vi "_word.table.Size.vi"(8 "error in (no error)":errorcluster, 11 "table Refnum in":refnum<k7>) -> (0 "error out":errorcluster, 1 "Cluster":cluster{"Row":i32, "Col":i32}, 3 "table Refnum out":refnum<k7>)   [LabVIEW 2018, in "WordReportGeneration.lvlib"]
uses:
  WordReportGeneration.lvlib
  <vilib>/Utility/NIReport.llb/NI_ReportGenerationCore.lvlib
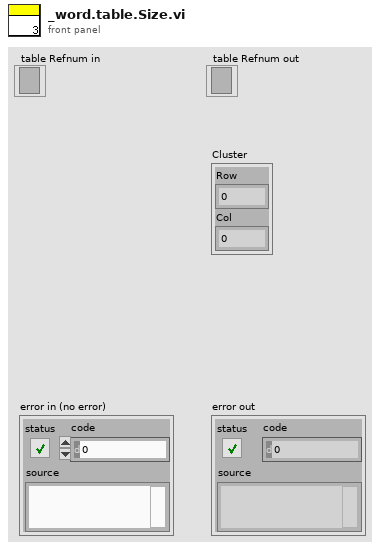
[diagram p1: front panel]
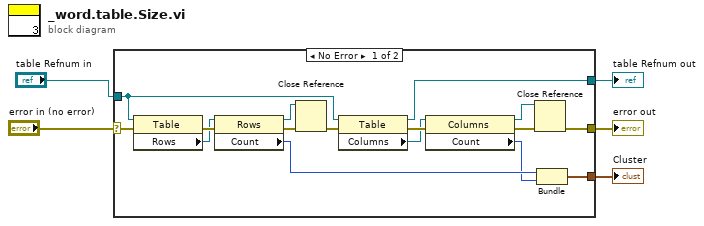
[diagram p0: block diagram]
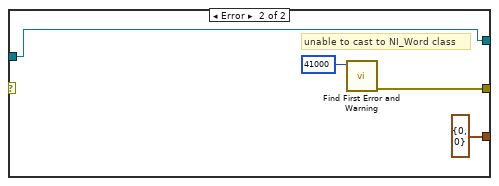
[diagram p2: hidden frame]
diagram:
  n1 = case shown="No Error" "error in (no error)" {
    selector: "error in (no error)" -> [w7 _]
    tunnel: [w15 w24] -> w5
    tunnel: "table Refnum in" -> [w14 w23]
    tunnel: [w21 w23] -> w2
    tunnel: [w20 cluster{"x+1":i32, i32} {"x+1"=0, 0}] -> w1
    frame No Error {
      n2 = property class="Table"(reference=w14, error in=w7) -> (error out=w13:errorcluster, "Rows"=w12:refnum<k7>)  [unwired: 1 out]
      n3 = property class="Rows"(reference=w12, error in=w13) -> (reference out=w10:refnum<k7>, error out=w11:errorcluster, "Count"=w9:i32)
      n4 = Close Reference(reference=w10, error in (no error)=w11) -> (error out=w6:errorcluster)
      n5 = property class="Table"(reference=w14, error in=w6) -> (reference out=w21:refnum<k7>, error out=w19:errorcluster, "Columns"=w18:refnum<k7>)
      n6 = property class="Columns"(reference=w18, error in=w19) -> (reference out=w16:refnum<k7>, error out=w17:errorcluster, "Count"=w8:i32)
      n7 = Close Reference(reference=w16, error in (no error)=w17) -> (error out=w15:errorcluster)
      n8 = Bundle("Count"=w9, "Count"=w8) -> (w20:cluster{"Count":i32, "Count":i32})  [unwired: 1 in]
    }
    frame Error {
      # "unable to cast to NI_Word class"
      n9 = call <vilib>:"Find First Error and Warning.vi"("error code"=41000) -> ("error out"=w24:errorcluster)  [unwired: 2 in, 4 out]
    }
  }
  "error out" <- w5
  "table Refnum out" <- w2
  "Cluster" <- w1
